vi "loadSocketFile.vi"(8 "error in (no error)":errorcluster, 9 "Machine":string, 11 "file path (use dialog)":path) -> (0 "error out":errorcluster)   [LabVIEW 2012]
uses:
  <vilib>/addons/database/Connection.llb/DB Tools Open Connec (Path).vi
  <vilib>/addons/database/Connection.llb/Conn Execute.vi
  <vilib>/addons/database/Recordset.llb/Rec Fetch Integer Data (R).vi
  <vilib>/addons/database/Recordset.llb/Rec Destroy - Connection.vi
  <vilib>/addons/database/NI_Database_API.lvlib
panel:
  out "text":string
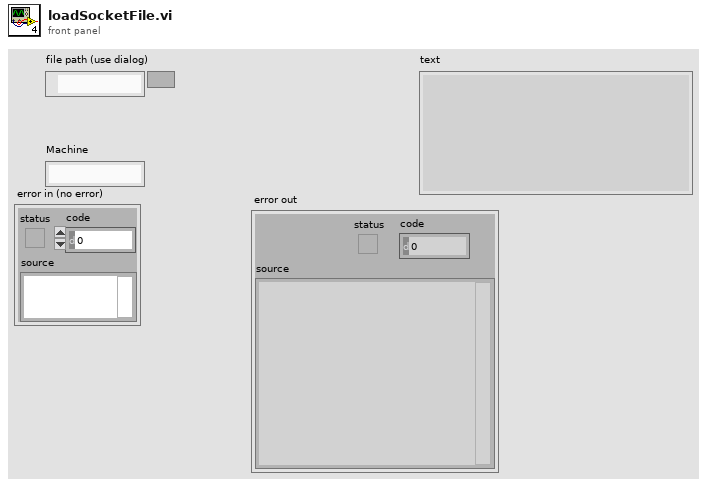
[diagram p1: front panel]
types:
  T1 = typedef "NI_Database_API.lvlib/Conn ObjectReference.ctl" = refnum<k1>
  T2 = typedef "NI_Database_API.lvlib/Rec ObjectReference.ctl" = refnum<k1>
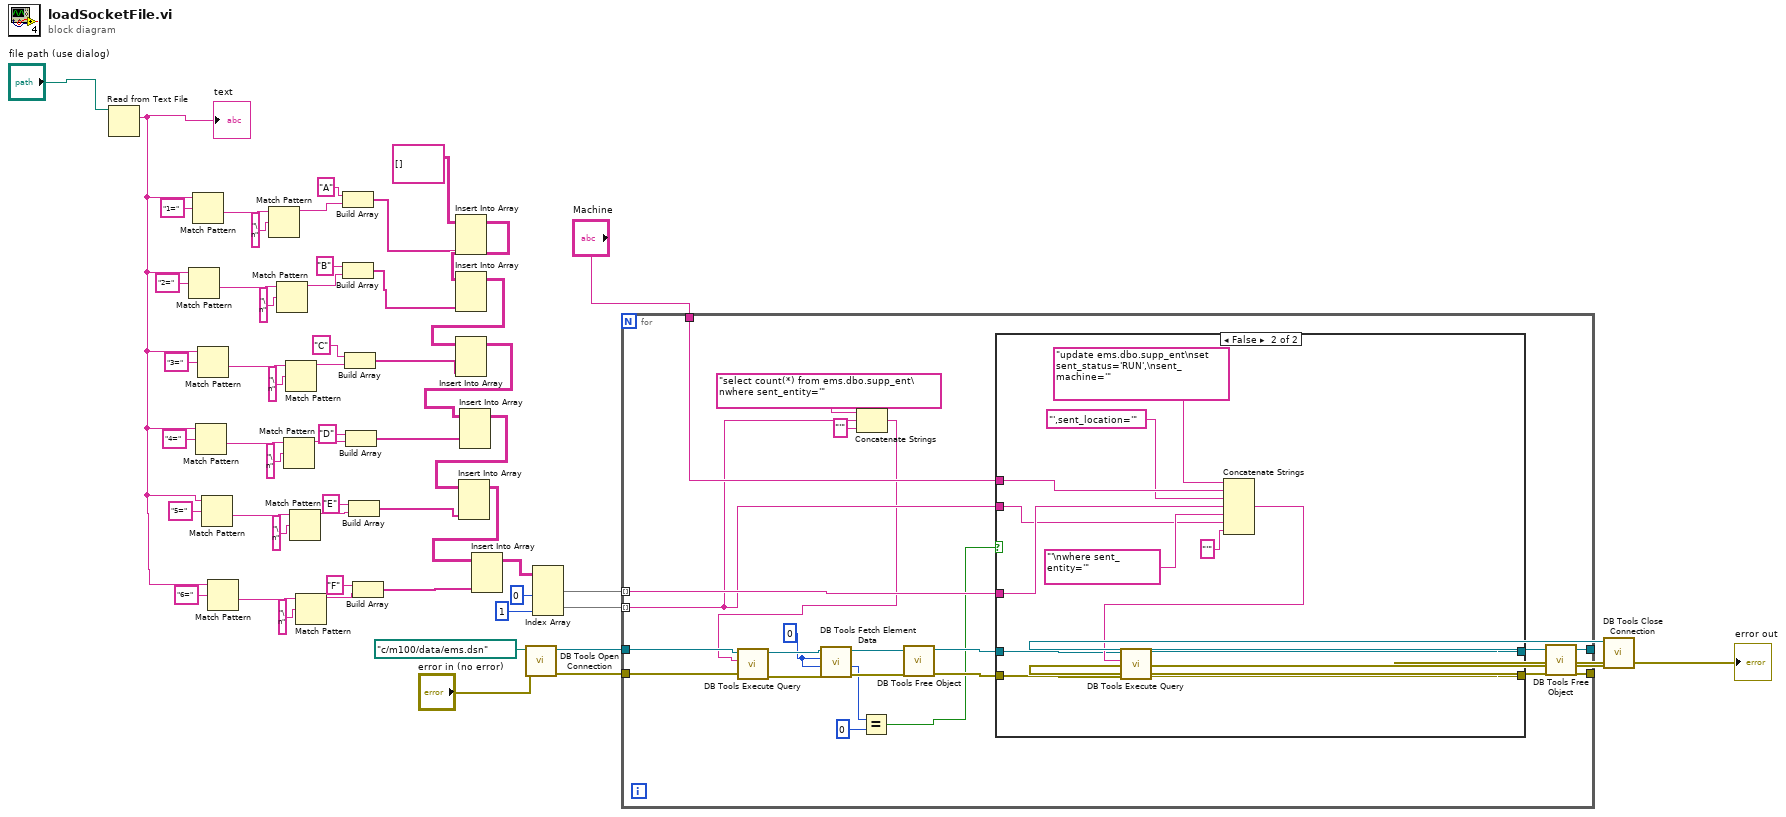
[diagram p0: block diagram]
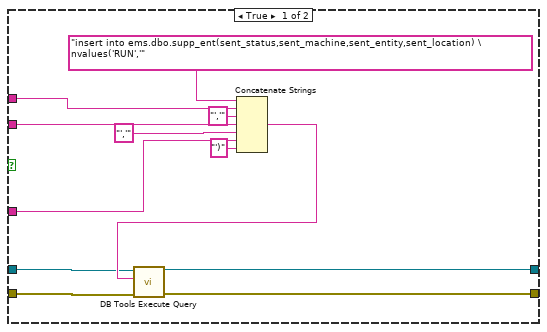
[diagram p2: hidden frame]
diagram:
  n1 = Read from Text File(file (use dialog)="file path (use dialog)") -> (text=w38:string)  [unwired: 3 in, 3 out]
  "text" <- w38
  n2 = Match Pattern(string=w38, regular expression="2=") -> (after substring=w52:string)  [unwired: 1 in, 3 out]
  n3 = Match Pattern(string=w38, regular expression="1=") -> (after substring=w55:string)  [unwired: 1 in, 3 out]
  n4 = Match Pattern(string=w38, regular expression="4=") -> (after substring=w46:string)  [unwired: 1 in, 3 out]
  n5 = Match Pattern(string=w38, regular expression="3=") -> (after substring=w49:string)  [unwired: 1 in, 3 out]
  n6 = Match Pattern(string=w38, regular expression="5=") -> (after substring=w43:string)  [unwired: 1 in, 3 out]
  n7 = Match Pattern(string=w38, regular expression="6=") -> (after substring=w40:string)  [unwired: 1 in, 3 out]
  n8 = Match Pattern(string=w55, regular expression="\n") -> (before substring=w27:string)  [unwired: 1 in, 3 out]
  n9 = Match Pattern(string=w52, regular expression="\n") -> (before substring=w24:string)  [unwired: 1 in, 3 out]
  n10 = Match Pattern(string=w46, regular expression="\n") -> (before substring=w18:string)  [unwired: 1 in, 3 out]
  n11 = Match Pattern(string=w49, regular expression="\n") -> (before substring=w21:string)  [unwired: 1 in, 3 out]
  n12 = Match Pattern(string=w43, regular expression="\n") -> (before substring=w15:string)  [unwired: 1 in, 3 out]
  n13 = Match Pattern(string=w40, regular expression="\n") -> (before substring=w11:string)  [unwired: 1 in, 3 out]
  n14 = Build Array("A" ("element"), w27) -> (w26:string[])
  n15 = Build Array("B" ("element"), w24) -> (w23:string[])
  n16 = Build Array("C" ("element"), w21) -> (w20:string[])
  n17 = Build Array("D" ("element"), w18) -> (w17:string[])
  n18 = Build Array("E" ("element"), w15) -> (w14:string[])
  n19 = Build Array("F" ("element"), w11) -> (w12:string[])
  n20 = Insert Into Array(array=string[][] [], new element=w26) -> (w32:string[][])  [unwired: 2 in]
  n21 = Insert Into Array(array=w32, new element=w23) -> (w31:string[][])  [unwired: 2 in]
  n22 = Insert Into Array(array=w31, new element=w20) -> (w30:string[][])  [unwired: 2 in]
  n23 = Insert Into Array(array=w30, new element=w17) -> (w29:string[][])  [unwired: 2 in]
  n24 = Insert Into Array(array=w29, new element=w14) -> (w28:string[][])  [unwired: 2 in]
  n25 = Insert Into Array(array=w28, new element=w12) -> (w9:string[][])  [unwired: 2 in]
  n26 = call-poly <vilib>:"DB Tools Open Connection.vi"("error in (no error)"="error in (no error)", "connection information"=path "c:/m100/data/ems.dsn") -> ("error out"=w35:errorcluster, "connection reference"=w37:T1)  [unwired: 6 in]
  n27 = Index Array(array=w9, index (col) #1=0 ("disabled index (col)"), index (col) #2=1 ("index (col)")) -> (element #1=w5:string[], element #2=w6:string[])  [unwired: 2 in]
  n28 = for {
    tunnel: w37 -> [w70]
    tunnel: [w78] -> w36
    tunnel: w35 -> [w69]
    tunnel: [w76] -> w34
    tunnel: w6 -> [w72] mode=indexing
    tunnel: w5 -> [w75] mode=indexing
    tunnel: "Machine" -> [w74]
    w61 = 0
    n29 = Concatenate Strings("select count(*) from ems.dbo.supp_ent\nwhere sent_entity='" ("string"), w72, "'" ("string")) -> (w62:string)
    n30 = call-poly <vilib>:"DB Tools Execute Query.vi"("error in (no error)"=w69, "SQL query"=w62, "connection reference"=w70) -> ("error out"=w64:errorcluster, "recordset reference"=w66:T2)  [unwired: 5 in]
    n31 = call-poly <vilib>:"DB Tools Fetch Element Data.vi"("error in (no error)"=w64, "type"=w61, "column index"=w61, "recordset reference"=w66) -> ("error out"=w63:errorcluster, "data"=w60:i32, "recordset reference out"=w65:T2)  [unwired: 3 in]
    n32 = Equal?(x=w60, y=0) -> (x = y?=w58:bool)
    n33 = call-poly <vilib>:"DB Tools Free Object.vi"("error in (no error)"=w63, "recordset reference"=w65) -> ("error out"=w67:errorcluster, "connection reference"=w68:T1)  [unwired: 8 in]
    n34 = case shown="False" w58 {
      tunnel: [w91 w103] -> w79
      tunnel: [w90 w102] -> w77
      tunnel: w75 -> [w88 w93]
      tunnel: w74 -> [w84 w97]
      tunnel: w72 -> [w82 w92]
      tunnel: w68 -> [w81 w95]
      tunnel: w67 -> [w80 w94]
      frame True {
        n35 = Concatenate Strings("insert into ems.dbo.supp_ent(sent_status,sent_machine,sent_entity,sent_location) \nvalues('RUN','" ("string"), w84, "','" ("string"), w82, "','" ("string"), w88, "')" ("string")) -> (w86:string)
        n36 = call-poly <vilib>:"DB Tools Execute Query.vi"("error in (no error)"=w80, "SQL query"=w86, "connection reference"=w81) -> ("error out"=w90:errorcluster, "recordset reference"=w91:T2)  [unwired: 5 in]
      }
      frame False {
        n37 = Concatenate Strings("update ems.dbo.supp_ent\nset sent_status='RUN',\nsent_machine='" ("string"), w97, "',sent_location='" ("string"), w93, "'\nwhere sent_entity='" ("string"), w92, "'" ("string")) -> (w99:string)
        n38 = call-poly <vilib>:"DB Tools Execute Query.vi"("error in (no error)"=w94, "SQL query"=w99, "connection reference"=w95) -> ("error out"=w102:errorcluster, "recordset reference"=w103:T2)  [unwired: 5 in]
      }
    }
    n39 = call-poly <vilib>:"DB Tools Free Object.vi"("error in (no error)"=w77, "recordset reference"=w79) -> ("error out"=w76:errorcluster, "connection reference"=w78:T1)  [unwired: 8 in]
  }
  n40 = call <vilib>:"DB Tools Close Connection.vi"("error in (no error)"=w34, "connection reference"=w36) -> ("error out"=→"error out":errorcluster)  [unwired: 5 in]
